vi "last_dcs_events_query.vi"(8 "error in (no error)":errorcluster, 10 "Limit":i32=2147483647, 11 "Min Time Stamp":timestamp) -> (0 "error out":errorcluster, 1 "No. of DCS 2 particles":i32, 2 "No. of DCS 1 particles":i32, 3 "DCS Array":dbl[][](array[numeric]))   [LabVIEW 2013]
uses:
  <vilib>/addons/database/_DB Variant To Data/Database Variant To Data.xnode
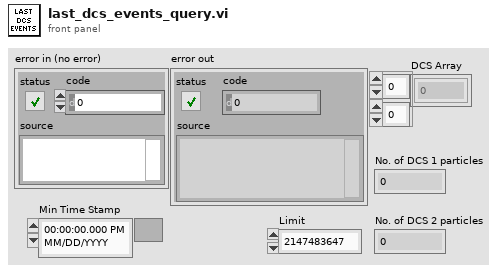
[diagram p1: front panel]
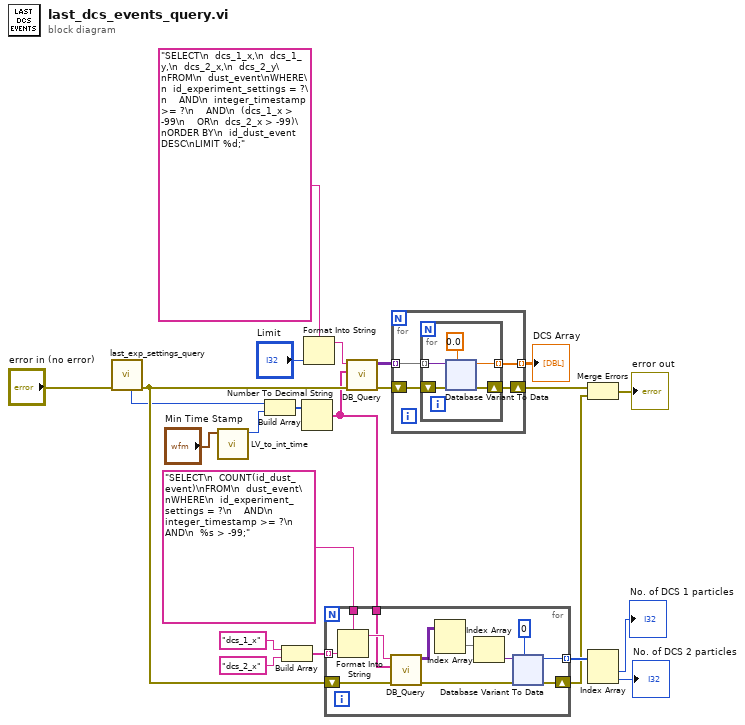
[diagram p0: block diagram]
diagram:
  n1 = call <userlib>:"last_exp_settings_query.vi"("error in (no error)"="error in (no error)") -> ("error out"=w9:errorcluster, "Experiment ID"=w1:i64)  [unwired: 5 in, 4 out]
  n2 = call <userlib>:"LV_to_int_time.vi"("Time Stamp"="Min Time Stamp") -> ("Integer Time"=w17:i64)  [unwired: 8 in, 1 out]
  n3 = Build Array(w1, w17) -> (w18:i64[])
  n4 = Build Array("dcs_1_x" ("input 1"), "dcs_2_x" ("input 1")) -> (w13:string[])
  n5 = Number To Decimal String(number=w18) -> (decimal integer string=w5:string[])  [unwired: 1 in]
  n6 = Format Into String(format string="SELECT\n  dcs_1_x,\n  dcs_1_y,\n  dcs_2_x,\n  dcs_2_y\nFROM\n  dust_event\nWHERE\n  id_experiment_settings = ?\n    AND\n  integer_timestamp >= ?\n    AND\n  (dcs_1_x > -99\n    OR\n  dcs_2_x > -99)\nORDER BY\n  id_dust_event DESC\nLIMIT %d;" ("Parameterized Query"), "Limit") -> (resulting string=w4:string)  [unwired: 2 in, 1 out]
  n7 = for {
    tunnel: "SELECT\n  COUNT(id_dust_event)\nFROM\n  dust_event\nWHERE\n  id_experiment_settings = ?\n    AND\n  integer_timestamp >= ?\n    AND\n  %s > -99;" ("Parameterized Query") -> [w34]
    tunnel: w13 -> [w33] mode=indexing
    tunnel: [w29] -> w12 mode=indexing
    shift-right: [w25] -> w7
    shift-left: w9 -> [w26]
    tunnel: w5 -> [w24]
    n8 = Format Into String(format string=w34, w33) -> (resulting string=w35:string)  [unwired: 2 in, 1 out]
    n9 = call <userlib>:"DB_Query.vi"("error in (no error)"=w26, "Parameters"=w24, "Parameterized Query"=w35) -> ("error out"=w31:errorcluster, "Results"=w32:variant[][])  [unwired: 6 in, 1 out]
    n10 = Index Array(array=w32) -> (element=w28:variant[])  [unwired: 2 in]
    n11 = Index Array(array=w28) -> (element=w27:variant)  [unwired: 1 in]
    n12 = xnode "Database Variant To Data"("database variant"=w27, "error in (no error)"=w31, "type"=0 ("index")) -> ("data"=w29:i32, "error out"=w25:errorcluster)
  }
  n13 = call <userlib>:"DB_Query.vi"("error in (no error)"=w9, "Parameters"=w5, "Parameterized Query"=w4) -> ("error out"=w21:errorcluster, "Results"=w22:variant[][])  [unwired: 6 in, 1 out]
  n14 = for {
    tunnel: w22 -> [w70] mode=indexing
    shift-right: [w68] -> w20
    shift-left: w21 -> [w71]
    tunnel: [w69] -> w19 mode=indexing
    n15 = for {
      shift-right: [w74] -> w68
      shift-left: w71 -> [w76]
      tunnel: w70 -> [w73] mode=indexing
      tunnel: [w72] -> w69 mode=indexing
      n16 = xnode "Database Variant To Data"("database variant"=w73, "error in (no error)"=w76, "type"=0.0) -> ("data"=w72:dbl, "error out"=w74:errorcluster)
    }
  }
  "DCS Array" <- w19
  n17 = Merge Errors(w20, w7) -> (→"error out":errorcluster)
  n18 = Index Array(array=w12) -> (element #1=→"No. of DCS 1 particles":i32, element #2=→"No. of DCS 2 particles":i32)  [unwired: 2 in]
